vi "Ping.vi"(6 "timeout (ms)":i32=5000, 8 "error in":errorcluster, 11 "gRPC ID in":T1) -> (0 "error out":errorcluster, 3 "gRPC ID out":T1)   [LabVIEW 2021, in "CIFManagerClientWrapper.lvlib"]
uses:
  <vilib>/gRPC/LabVIEW gRPC Library/Shared/grpcId.ctl
  CIF_Manager_client/RPC Messages/cif_manager_Empty.ctl
  CIFManagerClientWrapper.lvlib
  CIF_Manager_client/CIF_Manager_client.lvlib
  <vilib>/gRPC/LabVIEW gRPC Library/grpc-lvsupport-release.lvlib
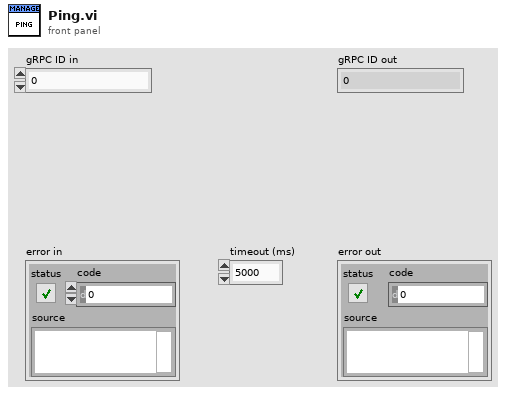
[diagram p1: front panel]
types:
  T1 = typedef "grpc-lvsupport-release.lvlib/grpcId.ctl" = u64
  T2 = typedef "CIF_Manager_client.lvlib/cif_manager_Empty.ctl" = cluster{"void":string}
  T3 = typedef "CIF_Manager_client.lvlib/cif_manager_Error.ctl" = cluster{"message":string, "code":i32}
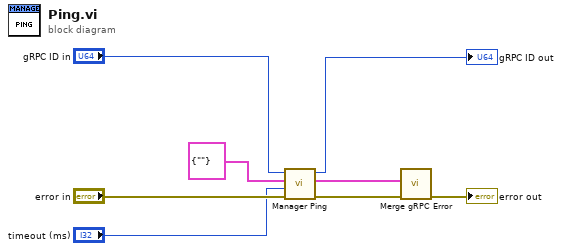
[diagram p0: block diagram]
diagram:
  n1 = call "Manager Ping.vi"("error in"="error in", "timeout (ms)"="timeout (ms)", "Request Data"=T2 {"void"=""}, "gRPC ID"="gRPC ID in") -> ("error out"=w4:errorcluster, "Response Data"=w2:T3, "gRPC ID out"=→"gRPC ID out":T1)  [unwired: 5 in]
  n2 = call "Merge gRPC Error.vi"("error in (no error)"=w4, "gRPC Error"=w2) -> ("error out"=→"error out":errorcluster)  [unwired: 9 in]
